vi "Load App.vi"(8 "error in (no error)":errorcluster, 11 "Status Notifier":refnum<notifier>) -> (0 "error out":errorcluster)   [LabVIEW 2013, in "Manager.lvlib" / "Manager.lvclass"]
doc: "Load the application into memory and start it running. The input notifier is used to send text to the splash screen to tell the user what stage the load process is in."
uses:
  Manager.lvclass
  PluginInterface/Actor Framework.lvlibp/Actor/Actor.lvclass
  PluginInterface/Actor Framework.lvlibp/Message Queue/Message Queue.lvclass
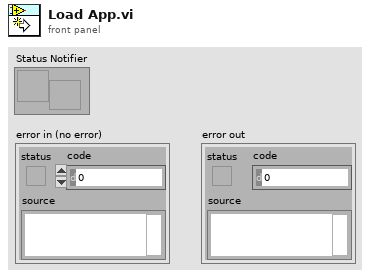
[diagram p1: front panel]
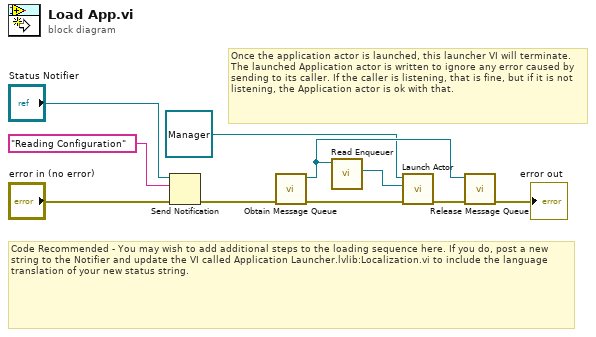
[diagram p0: block diagram]
diagram:
  # "Once the application actor is launched, this launcher VI will terminate. The launched Application actor is written to ignore any error caused by sending to its caller. If the caller is listening, that is fine, but if it is not listening, the Application actor is ok with that."
  # "Code Recommended - You may wish to add additional steps to the loading sequence here. If you do, post a new string to the Notifier and update the VI called Application Launcher.lvlib:Localization.vi to include the language translation of your new status string."
  n1 = Send Notification(notification="Reading Configuration", notifier="Status Notifier", error in (no error)="error in (no error)") -> (error out=w2:errorcluster)  [unwired: 1 out]
  n2 = call "Obtain Message Queue.vi"("error in (no error)"=w2) -> ("error out"=w4:errorcluster, "Message Queue"=w3:refnum<class "Message Queue.lvclass">)  [unwired: 9 in]
  n3 = call "Read Enqueuer.vi"("Message Queue"=w3) -> ("Message Enqueuer"=w7:refnum<class "Message Enqueuer.lvclass">)  [unwired: 10 in]
  n4 = call "Launch Actor.vi"("error in (no error)"=w4, "Actor-to-Caller Enqueuer"=w7, "Actor"=refnum<class "Manager.lvclass"> refnum ("My Application.lvclass")) -> ("error out"=w6:errorcluster)  [unwired: 7 in, 1 out]
  n5 = call "Release Message Queue.vi"("error in (no error)"=w6, "Message Queue"=w3) -> ("error out"=→"error out":errorcluster)  [unwired: 8 in, 1 out]
